vi "oax_gsGet Selected Item Name in Listbox.vi"(2 "error in (no error)":errorcluster, 3 "ctrl reference":refnum<vi>) -> (0 "error out":errorcluster, 1 "selected item":string)   [LabVIEW 2017]
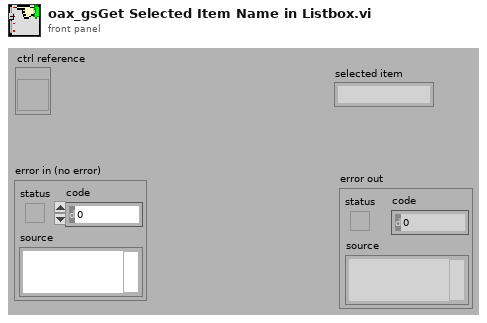
[diagram p1: front panel]
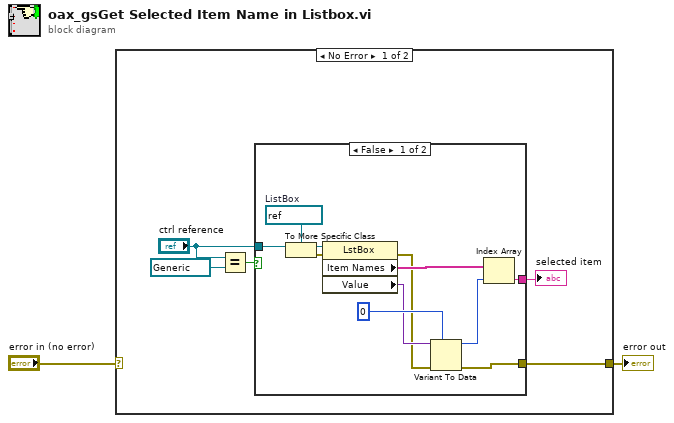
[diagram p0: block diagram]
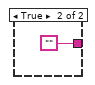
[diagram p2: hidden frame]
diagram:
  n1 = case shown="No Error" "error in (no error)" {
    selector: "error in (no error)" -> [_ w20]
    tunnel: [w7 w20] -> w1
    frame No Error {
      n2 = Equal?(x="ctrl reference", y=refnum<vi> refnum) -> (x = y?=w5:bool)
      n3 = case shown="False" w5 {
        tunnel: [w11 _] -> w7
        tunnel: [w9 ""] -> w6
        tunnel: "ctrl reference" -> [w8 _]
        frame False {
          w18 = refnum<vi> refnum  # ListBox
          n4 = To More Specific Class(target class=w18, reference=w8) -> (specific class reference=w16:refnum<vi>, error out=w17:errorcluster)  [unwired: 1 in]
          n5 = property class="LstBox"(reference=w16, error in=w17) -> (error out=w12:errorcluster, "Item Names"=w15:string[], "Value"=w13:variant)  [unwired: 1 out]
          n6 = Variant To Data(error in=w12, type=0, Variant=w13) -> (data=w10:i32, error out=w11:errorcluster)
          n7 = Index Array(array=w15, index=w10) -> (element=w9:string)
        }
        frame True {
        }
      }
      "selected item" <- w6
    }
    frame Error {
    }
  }
  "error out" <- w1
